vi "AutoEnd.vi"(1 "Time Since Latch":u32, 2 "Instruction String":string) -> (0 "Advance Trigger":bool)   [LabVIEW 2019]
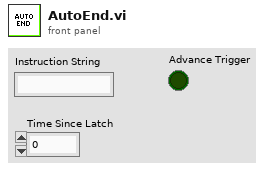
[diagram p1: front panel]
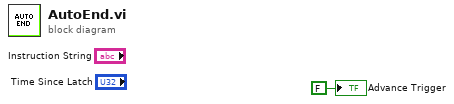
[diagram p0: block diagram]
diagram:
  "Advance Trigger" <- FALSE ("Advance Trigger")
